vi "Hello World.vi"() -> ()   [LabVIEW 2017]
panel:
  in  "Message":string="Hello World!"
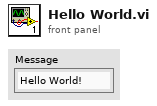
[diagram p1: front panel]
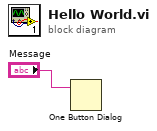
[diagram p0: block diagram]
diagram:
  n1 = One Button Dialog(message="Message") -> ()  [unwired: 1 in, 1 out]
